vi "ProductCount.vi"(6 "DUT":i32, 7 "instrument file path":path, 8 "error in (no error)":errorcluster, 9 "Init":bool, 10 "Key_name":string[](array[string])=["Total Run", "Pass", "Fail"], 11 "Part Count":T1) -> (0 "error out":errorcluster, 2 "Part Count  2":T1)   [LabVIEW 2024, in "Test_2.lvlib"]
uses:
  Test_2.lvlib
  Launcher/Launcher_DTU.lvlib
  Launcher/SubVI/Controls/OEE_CTRL.ctl
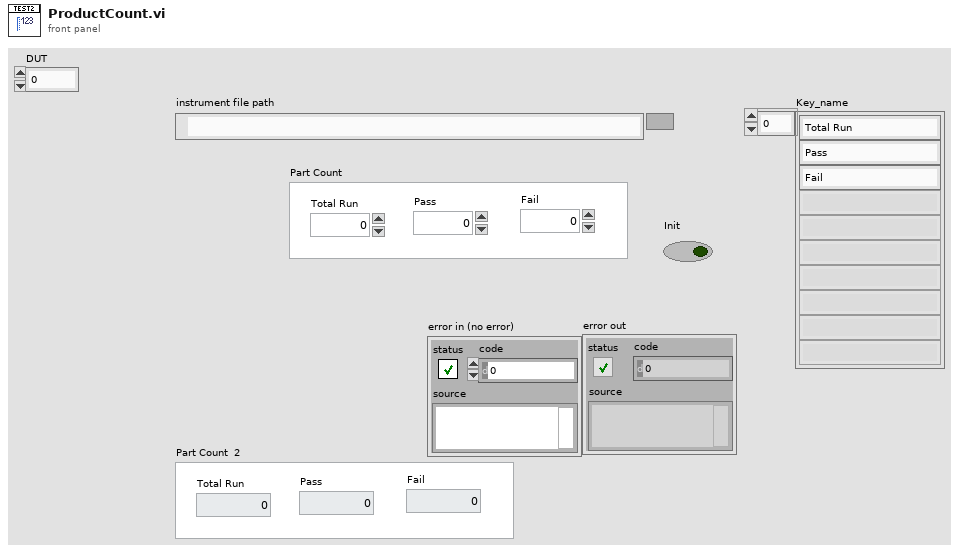
[diagram p1: front panel]
types:
  T1 = typedef "Launcher_DTU.lvlib/OEE_CTRL.ctl" = cluster{"Total Run":i32, "Pass":i32, "Fail":i32}
  T2 = enum16{"Read", "Write", "All_sections", "All_values", "Remove key&section"}
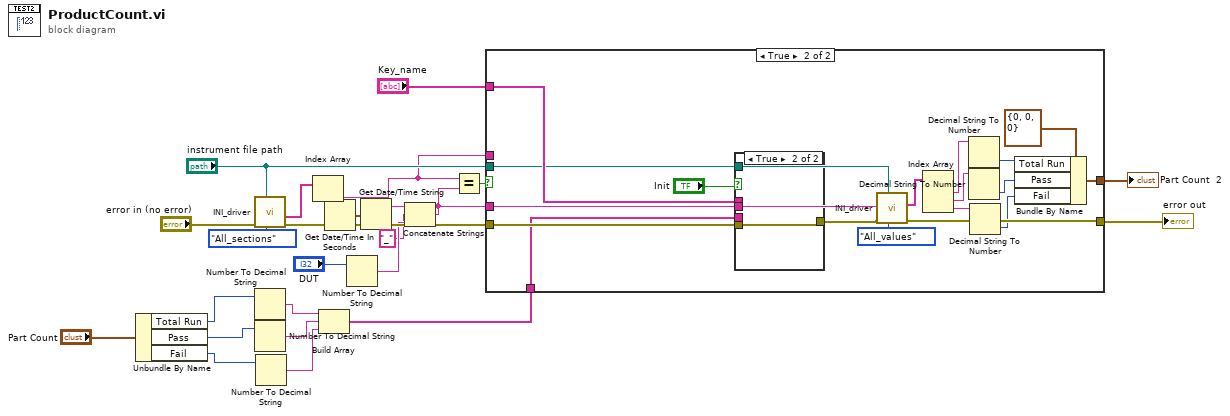
[diagram p0: block diagram]
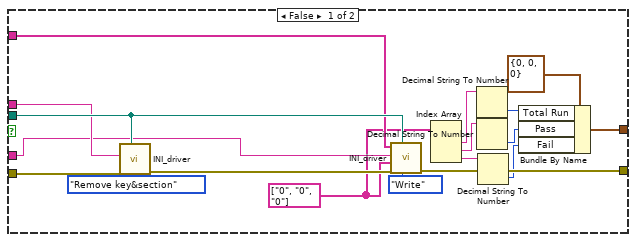
[diagram p2: hidden frame]
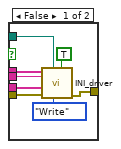
[diagram p3: hidden frame]
diagram:
  n1 = Unbundle By Name("Part Count") -> ("Total Run"=w12:i32, "Pass"=w11:i32, "Fail"=w10:i32)
  n2 = call "INI_driver.vi"("Enum"=T2."All_sections", "instrument file path"="instrument file path", "error in (no error)"="error in (no error)") -> ("error out"=w23:errorcluster, "section names"=w20:string[])  [unwired: 5 in, 2 out]
  n3 = Number To Decimal String(number=w12) -> (decimal integer string=w7:string)  [unwired: 1 in]
  n4 = Number To Decimal String(number=w11) -> (decimal integer string=w8:string)  [unwired: 1 in]
  n5 = Number To Decimal String(number=w10) -> (decimal integer string=w9:string)  [unwired: 1 in]
  n6 = Index Array(array=w20) -> (element=w15:string)  [unwired: 1 in]
  n7 = Build Array(w7, w8, w9) -> (w6:string[])
  n8 = Get Date/Time In Seconds() -> (seconds since 1Jan1904=w24:timestamp)
  n9 = Number To Decimal String(number="DUT") -> (decimal integer string=w2:string)  [unwired: 1 in]
  n10 = Get Date/Time String(seconds (now)=w24) -> (date string=w14:string)  [unwired: 2 in, 1 out]
  n11 = Concatenate Strings(w14, "_" ("string"), w2) -> (w3:string)
  n12 = Equal?(x=w15, y=w3) -> (x = y?=w19:bool)
  n13 = case shown="True" w19 {
    tunnel: w23 -> [w39 w60]
    tunnel: "instrument file path" -> [w38 w54]
    tunnel: w3 -> [w34 w53]
    tunnel: "Key_name" -> [w37 w59]
    tunnel: w6 -> [_ w58]
    tunnel: [w36 w56] -> w16
    tunnel: w15 -> [w35 _]
    tunnel: [w32 w51] -> w5
    frame False {
      w28 = string[] ["0", "0", "0"] ("Value_in")
      n14 = call "INI_driver.vi"("Enum"=T2."Remove key&section", "instrument file path"=w38, "error in (no error)"=w39, "Section"=w35) -> ("error out"=w41:errorcluster)  [unwired: 4 in, 3 out]
      n15 = call "INI_driver.vi"("Enum"=T2."Write", "instrument file path"=w38, "error in (no error)"=w41, "Value_in"=w28, "Section"=w34, "Key_name"=w37) -> ("error out"=w36:errorcluster)  [unwired: 2 in, 3 out]
      n16 = Index Array(array=w28) -> (element #1=w31:string, element #2=w30:string, element #3=w29:string)  [unwired: 3 in]
      n17 = Decimal String To Number(string=w31) -> (number=w25:i32)  [unwired: 2 in, 1 out]
      n18 = Decimal String To Number(string=w30) -> (number=w26:i32)  [unwired: 2 in, 1 out]
      n19 = Decimal String To Number(string=w29) -> (number=w27:i32)  [unwired: 2 in, 1 out]
      n20 = Bundle By Name(cluster=T1 {"Total Run"=0, "Pass"=0, "Fail"=0} ("Part Count  2"), "Total Run"=w25, "Pass"=w26, "Fail"=w27) -> (w32:T1)
    }
    frame True {
      n21 = case shown="True" "Init" {
        tunnel: w60 -> [w68 w69]
        tunnel: w59 -> [w66 _]
        tunnel: w58 -> [w65 _]
        tunnel: [w64 w69] -> w57
        tunnel: w54 -> [w63 _]
        tunnel: w53 -> [w62 _]
        frame False {
          n22 = call "INI_driver.vi"("create file if necessary (T)"=TRUE, "Enum"=T2."Write", "instrument file path"=w63, "error in (no error)"=w68, "Value_in"=w65, "Section"=w62, "Key_name"=w66) -> ("error out"=w64:errorcluster)  [unwired: 1 in, 3 out]
        }
        frame True {
        }
      }
      n23 = call "INI_driver.vi"("Enum"=T2."All_values", "instrument file path"=w54, "error in (no error)"=w57, "Section"=w53) -> ("error out"=w56:errorcluster, "Values out"=w50:string[])  [unwired: 4 in, 2 out]
      n24 = Index Array(array=w50) -> (element #1=w48:string, element #2=w47:string, element #3=w45:string)  [unwired: 3 in]
      n25 = Decimal String To Number(string=w48) -> (number=w49:i32)  [unwired: 2 in, 1 out]
      n26 = Decimal String To Number(string=w47) -> (number=w46:i32)  [unwired: 2 in, 1 out]
      n27 = Decimal String To Number(string=w45) -> (number=w44:i32)  [unwired: 2 in, 1 out]
      n28 = Bundle By Name(cluster=T1 {"Total Run"=0, "Pass"=0, "Fail"=0} ("Part Count  2"), "Total Run"=w49, "Pass"=w46, "Fail"=w44) -> (w51:T1)
    }
  }
  "error out" <- w16
  "Part Count  2" <- w5
